vi "to_xml.vi"(8 "error in":errorcluster, 11 "Variable Settings":T1={"Measurements per Iteration"=1, "Local Data Path"=path "C:/Users/Saffmanlab/Documents/Cesium/data", "Experiment description suffix for filename (no spaces please)"="", "Network Data Path"=path "Z:/", "Copy data to network"=TRUE, "Measurement Timeout (ms)"=0, "Independent Variables"=[], "Dependent Variables"=[], "Run Test Mode"=FALSE} {"Independent Variables"."# steps" min=1 step=1; "Measurements per Iteration" min=1 step=1}) -> (0 "error out":errorcluster, 3 "varible settings string":string)   [LabVIEW 2012, in "ExperimentVariables.lvclass"]
doc: "Saves experiment variable settings in the format:\n\n<IndependentVariables columns=\"Description,Name (a,a0...a9),min,max,# steps\">\n<var>%s\\t%s\\t%f\\t%f\\t%u</var>\n</IndependentVariables>\n<DependentVariables columns=\"Description,Name (a,a0...a9),Equation,Result\">\n<var>%s\\t%s\\t%s\\t%f</var>\n</DependentVariables>\n<MeasurementsPerIteration>%u</MeasurementsPerIteration>\n<LocalDataPath>%s</LocalDataPath>\n<ExperimentDescriptionSuffix>%s</ExperimentDescriptionSuffix>\n<NetworkDataPath>%s</NetworkDataPath>\n<CopyDataToNetwork>%b</CopyDataToNetwork>\n<MeasurementTimeout units=\"ms\">%u</MeasurementTimeout>\n<RunTestMode>%b</RunTestMode>\n\nMTL 2013 Jan 1"
uses:
  ExperimentVariables.lvclass
  Variable_Settings.ctl
panel:
  # "Parameters will be evaluated once at the beginning of the experiment from top to bottom, \nso any parameter may depend on all those above it.\nVariables will be evaluated each iteration.\nParameters and Variables may be used in various other experiment settings, as noted.\nSee LabView Help -> Formula Node and Expression Node Functions for a list of available functions."
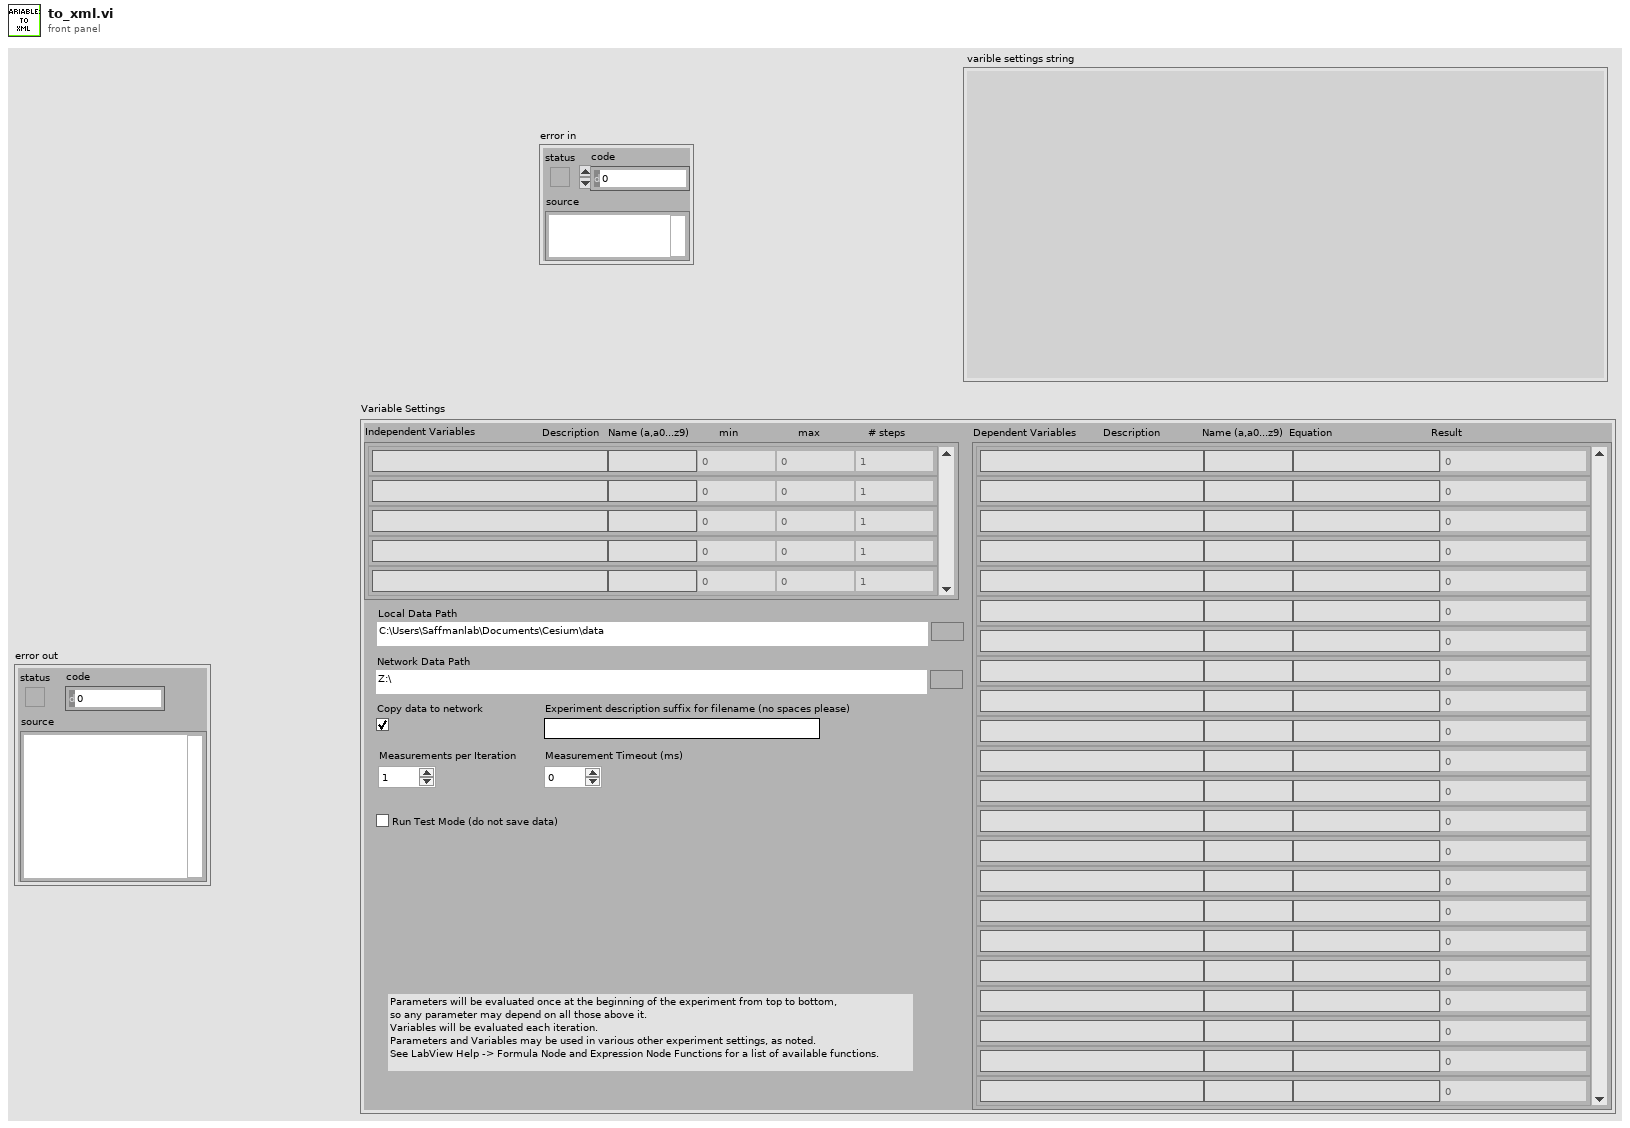
[diagram p1: front panel]
types:
  T1 = typedef "ExperimentVariables.lvclass/Variable_Settings.ctl" = cluster{"Measurements per Iteration":i32, "Local Data Path":path, "Experiment description suffix for filename (no spaces please)":string, "Network Data Path":path, "Copy data to network":bool, "Measurement Timeout (ms)":u32, "Independent Variables":cluster{"Description":string, "Name (a,a0...a9)":string, "min":dbl, "max":dbl, "# steps":u32}[], "Dependent Variables":cluster{"Description":string, "Name (a,a0...a9)":string, "Equation":string, "Result":dbl}[], "Run Test Mode":bool}
  T2 = cluster{"Description":string, "Name (a,a0...a9)":string, "min":dbl, "max":dbl, "# steps":u32}[]
  T3 = cluster{"Description":string, "Name (a,a0...a9)":string, "Equation":string, "Result":dbl}[]
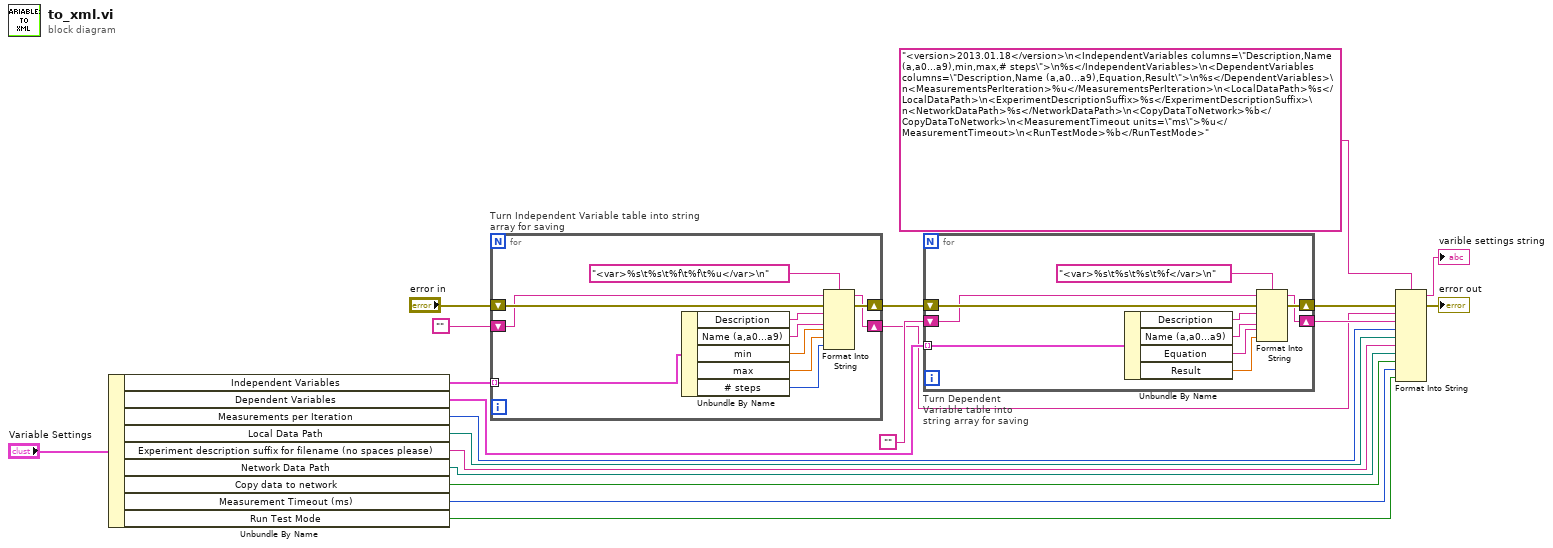
[diagram p0: block diagram]
diagram:
  n1 = Unbundle By Name("Variable Settings") -> ("Independent Variables"=w4:T2, "Dependent Variables"=w3:T3, "Measurements per Iteration"=w8:i32, "Local Data Path"=w19:path, "Experiment description suffix for filename (no spaces please)"=w18:string, "Network Data Path"=w17:path, "Copy data to network"=w16:bool, "Measurement Timeout (ms)"=w15:u32, "Run Test Mode"=w7:bool)
  n2 = for "Turn Independent Variable table into string array for saving" {
    tunnel: w4 -> [w24] mode=indexing
    shift-right: [w27] -> w20
    shift-left: "error in" -> [w28]
    shift-right: [w26] -> w1
    shift-left: "" -> [w21]
    n3 = Unbundle By Name(w24) -> ("Description"=w22:string, "Name (a,a0...a9)"=w23:string, "min"=w30:dbl, "max"=w29:dbl, "# steps"=w25:u32)
    n4 = Format Into String(format string="<var>%s\t%s\t%f\t%f\t%u</var>\n", initial string=w21, error in=w28, w22, w23, w30, w29, w25) -> (resulting string=w26:string, error out=w27:errorcluster)
  }
  n5 = for "Turn Dependent Variable table into string array for saving" {
    tunnel: w3 -> [w41] mode=indexing
    shift-right: [w36] -> w13
    shift-left: w20 -> [w37]
    shift-right: [w35] -> w2
    shift-left: "" -> [w32]
    n6 = Unbundle By Name(w41) -> ("Description"=w33:string, "Name (a,a0...a9)"=w34:string, "Equation"=w39:string, "Result"=w38:dbl)
    n7 = Format Into String(format string="<var>%s\t%s\t%s\t%f</var>\n", initial string=w32, error in=w37, w33, w34, w39, w38) -> (resulting string=w35:string, error out=w36:errorcluster)
  }
  n8 = Format Into String(format string="<version>2013.01.18</version>\n<IndependentVariables columns=\"Description,Name (a,a0...a9),min,max,# steps\">\n%s</IndependentVariables>\n<DependentVariables columns=\"Description,Name (a,a0...a9),Equation,Result\">\n%s</DependentVariables>\n<MeasurementsPerIteration>%u</MeasurementsPerIteration>\n<LocalDataPath>%s</LocalDataPath>\n<ExperimentDescriptionSuffix>%s</ExperimentDescriptionSuffix>\n<NetworkDataPath>%s</NetworkDataPath>\n<CopyDataToNetwork>%b</CopyDataToNetwork>\n<MeasurementTimeout units=\"ms\">%u</MeasurementTimeout>\n<RunTestMode>%b</RunTestMode>", error in=w13, w1, w2, w8, w19, w18, w17, w16, w15, w7) -> (resulting string=→"varible settings string":string, error out=→"error out":errorcluster)  [unwired: 1 in]
